vi "transmit additional endpoints.vi"(11 "Oauth2":refnum<class "Oauth2.lvclass">) -> (2 "Additional Endpoints":string[](array[string]))   [LabVIEW 2013, in "Oauth2.lvclass"]
uses:
  Oauth2.lvclass
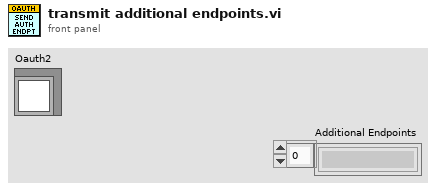
[diagram p1: front panel]
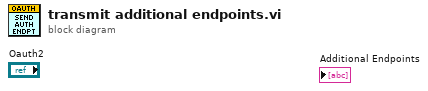
[diagram p0: block diagram]
diagram:
